vi "_Find Cell.vi"(8 "error in":errorcluster, 9 "Lexical Index":string, 10 "Row":refnum<k24>) -> (0 "error out":errorcluster, 2 "Cell":refnum<k24>)   [LabVIEW 2021, in "Open Xml.lvlib"]
uses:
  Open Xml.lvlib
  D:/git/Open-Xml-LabVIEW/DocumentFormat.OpenXml.dll
  DocumentFormat.OpenXml.dll
  D:/git/Open-Xml-LabVIEW/DocumentFormat.OpenXml.Framework.dll
  DocumentFormat.OpenXml.Framework.dll
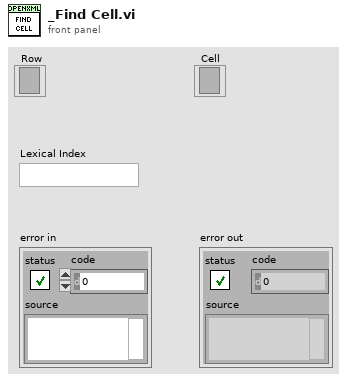
[diagram p1: front panel]
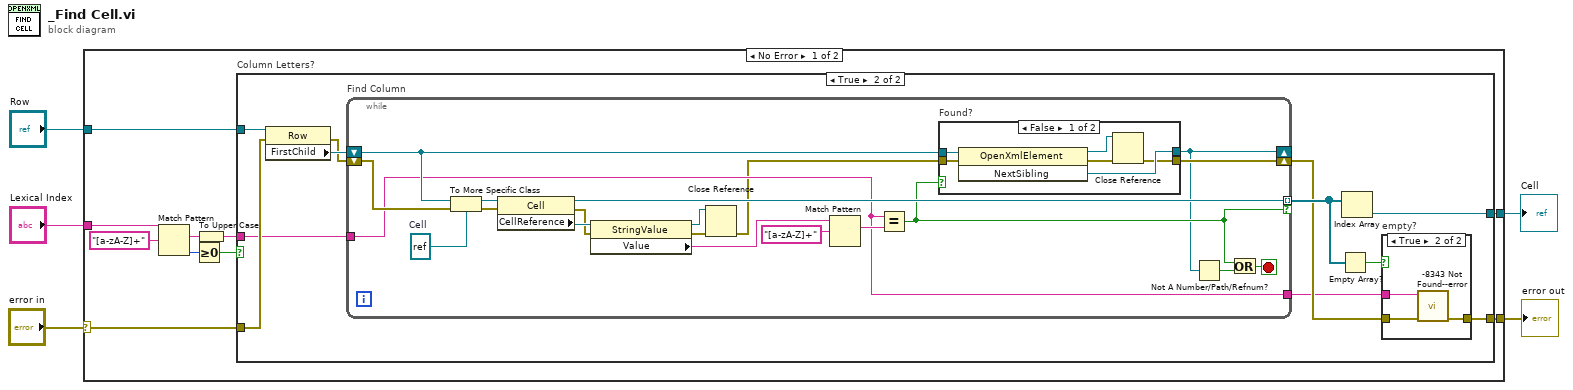
[diagram p0: block diagram]
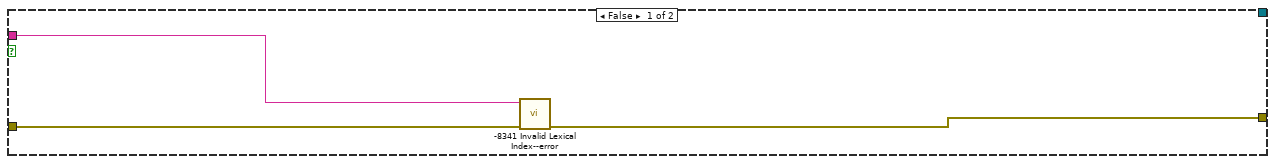
[diagram p2: hidden frame]
diagram:
  n1 = case shown="No Error" "error in" {
    selector: "error in" -> [w14 w62]
    tunnel: "Row" -> [w15 _]
    tunnel: "Lexical Index" -> [w12 _]
    tunnel: [w9 w62] -> w2
    tunnel: [w8 _] -> w1
    frame No Error {
      n2 = Match Pattern(string=w12, regular expression="[a-zA-Z]+") -> (match substring=w11:string, offset past match=w10:i32)  [unwired: 1 in, 2 out]
      n3 = Greater Or Equal To 0?(x=w10) -> (x >= 0?=w7:bool)
      n4 = To Upper Case(1:w11) -> (0:w6:string)
      n5 = case "Column Letters?" shown="True" w7 {
        tunnel: w15 -> [_ w29]
        tunnel: w14 -> [w18 w28]
        tunnel: w6 -> [w16 w25]
        tunnel: [w17 w19] -> w9
        tunnel: [_ w24] -> w8
        frame False {
          n6 = call "-8341 Invalid Lexical Index--error.vi"("error in"=w18, "Lexical Index"=w16) -> ("error out"=w17:errorcluster)  [unwired: 9 in]
        }
        frame True {
          n7 = property class="Row"(reference=w29, error in=w28) -> (error out=w26:errorcluster, "FirstChild"=w27:refnum<k24>)  [unwired: 1 out]
          n8 = while "Find Column" {
            shift-right: [w47] -> w21
            shift-left: w26 -> [w53]
            shift-right: [w38] -> _
            shift-left: w27 -> [w37]
            tunnel: [w49] -> w23 mode=indexing if=w39
            tunnel: w25 -> [w36]
            tunnel: [w36] -> w20
            stop <- w51 stop-if-true
            w46 = refnum<k24> refnum  # Cell
            n9 = To More Specific Class(target class=w46, reference=w37, error in=w53) -> (specific class reference=w50:refnum<k24>, error out=w48:errorcluster)
            n10 = property class="Cell"(reference=w50, error in=w48) -> (reference out=w49:refnum<k24>, error out=w43:errorcluster, "CellReference"=w45:refnum<k24>)
            n11 = property class="StringValue"(reference=w45, error in=w43) -> (reference out=w34:refnum<k24>, error out=w44:errorcluster, "Value"=w41:string)
            n12 = Close Reference(reference=w34, error in (no error)=w44) -> (error out=w35:errorcluster)
            n13 = Match Pattern(string=w41, regular expression="[a-zA-Z]+") -> (match substring=w40:string)  [unwired: 1 in, 3 out]
            n14 = Equal?(x=w36, y=w40) -> (x = y?=w39:bool)
            n15 = case "Found?" shown="False" w39 {
              tunnel: [w55 w60] -> w47
              tunnel: w37 -> [w58 w61]
              tunnel: [w56 w61] -> w38
              tunnel: w35 -> [w57 w60]
              frame False {
                n16 = invoke class="OpenXmlElement" method="NextSibling"(reference=w58, error in=w57) -> (reference out=w54:refnum<k24>, error out=w59:errorcluster, "NextSibling"=w56:refnum<k24>)  [unwired: 1 in]
                n17 = Close Reference(reference=w54, error in (no error)=w59) -> (error out=w55:errorcluster)
              }
              frame True {
              }
            }
            n18 = Not A Number/Path/Refnum?(number/path/refnum=w38) -> (NaN/Path/Refnum?=w52:bool)
            n19 = Or(x=w39, y=w52) -> (x .or. y?=w51:bool)
          }
          n20 = Empty Array?(array=w23) -> (empty?=w22:bool)
          n21 = Index Array(array=w23) -> (element=w24:refnum<k24>)  [unwired: 1 in]
          n22 = case "empty?" shown="True" w22 {
            tunnel: w21 -> [w30 w33]
            tunnel: w20 -> [_ w32]
            tunnel: [w30 w31] -> w19
            frame False {
            }
            frame True {
              n23 = call "-8343 Not Found--error.vi"("error in (no error)"=w33, "Item"=w32) -> ("error out"=w31:errorcluster)  [unwired: 9 in]
            }
          }
        }
      }
    }
    frame Error {
    }
  }
  "error out" <- w2
  "Cell" <- w1
